vi "Update Task List.vi"(8 "error in (no error)":errorcluster, 11 "BuildWorker in":refnum<class "BuildWorker.lvclass">) -> (0 "error out":errorcluster, 3 "BuildWorker out":refnum<class "BuildWorker.lvclass">)   [LabVIEW 2017, in "BuildWorker.lvlib" / "BuildWorker.lvclass"]
uses:
  BuildWorker.lvclass
  BuildWorker.lvclass/BuildWorker.ctl
  Classes/Task/Task.lvclass/Task.ctl
  Classes/Task/Get Name.vi
  Classes/Task/Get Status String.vi
  Classes/Task/Task.lvclass
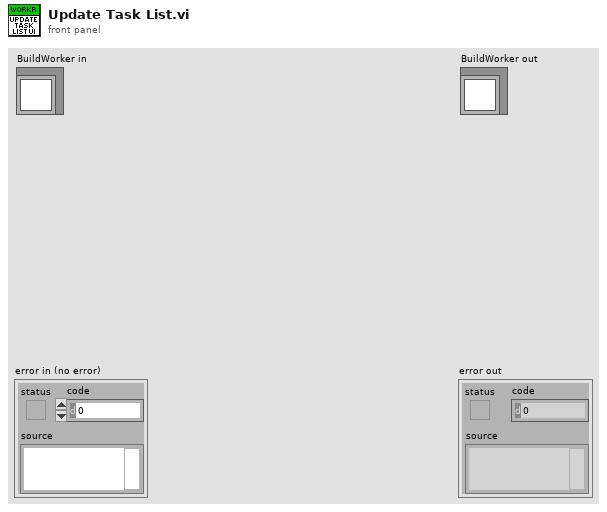
[diagram p1: front panel]
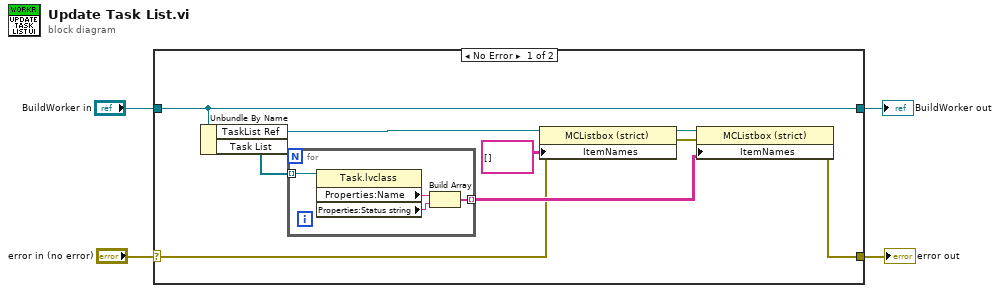
[diagram p0: block diagram]
diagram:
  n1 = case shown="No Error" "error in (no error)" {
    selector: "error in (no error)" -> [w6 w19]
    tunnel: [w5 w19] -> w3
    tunnel: [w13 w18] -> w1
    tunnel: "BuildWorker in" -> [w13 w18]
    frame No Error {
      n2 = Unbundle By Name(w13) -> ("TaskList Ref"=w11:refnum<vi>, "Task List"=w12:refnum<class "Task.lvclass">[])
      n3 = for {
        tunnel: w12 -> [w17] mode=indexing
        tunnel: [w14] -> w9 mode=indexing
        n4 = property class="Task.lvclass"(reference=w17) -> ("Properties:Name"=w16:string, "Properties:Status string"=w15:string)  [unwired: 1 in, 2 out]
        n5 = Build Array(w16, w15) -> (w14:string[])
      }
      n6 = property class="MCListbox (strict)"(reference=w11, error in=w6, "ItemNames"=string[][] [] ("Item Names")) -> (reference out=w10:refnum<vi>, error out=w7:errorcluster)
      n7 = property class="MCListbox (strict)"(reference=w10, error in=w7, "ItemNames"=w9) -> (error out=w5:errorcluster)  [unwired: 1 out]
    }
    frame Error {
    }
  }
  "error out" <- w3
  "BuildWorker out" <- w1
